vi "complexsignalpropogation.vi"() -> ()   [LabVIEW 2009]
uses:
  <vilib>/imath/engines/lvmath2/RunTimeEngine/ErrorHandling/NIMS_Finalize Error.vi
  <vilib>/imath/engines/lvmath2/RunTimeEngine/Parser/MC_Version.vi
  <vilib>/imath/engines/lvmath2/RunTimeEngine/Managers/WorkSpace/UID Generator.vi
  <vilib>/imath/engines/lvmath2/RunTimeEngine/NodeEndStatement/NIMS_NodeEndStatement_Output.vi
  <instcachedir>/0/NIMS_NodeEndStatement_Output_53EC0D466D134D7ABD903AC30B43404B.lvgen/NIMS_NodeEndStatement_Output_53EC0D466D134D7ABD903AC30B43404B_001.vi
  <vilib>/imath/engines/lvmath2/RunTimeEngine/NodeEndStatement/MC_NodeEndStatement_Dispose.vi
  <vilib>/imath/engines/lvmath/Functions/Error Handling/MergeErrorsWrapper.vi
  <vilib>/imathl/engines/lvmath/Functions/Error Handling/Create Error.vi
  <vilib>/imath/engines/lvmath2/RunTimeEngine/RunTimeType/NIMS_RunTimeType_Get Case Value.vi
  <vilib>/imath/engines/lvmath2/RunTimeEngine/Managers/SymbolTable/Read Variable.vi
  <vilib>/imath/engines/lvmath2/RunTimeEngine/CommandStatement/NIMS_CommandStatement_MaskErr.vi
  <vilib>/imath/engines/lvmath2/RunTimeEngine/Managers/SymbolTable/Write Variable.vi
  <vilib>/imath/engines/lvmath2/RunTimeEngine/ArithmeticOperatorToken/NIMS_NS_ArithmeticOperator_cctranspose.vi
  <vilib>/imath/engines/lvmath2/RunTimeEngine/RunTimeSymbolToken/NIMS_RunTimeSymbolToken_ReadVariable.vi
  <vilib>/imath/engines/lvmath2/RunTimeEngine/RangeToken/NIMS_NS_Range - 2 inputs.vi
  <vilib>/imath/engines/lvmath2/RunTimeEngine/RunTimeSymbolToken/NIMS_RunTimeSymbolToken_ResolveSymbol.vi
  <instcachedir>/0/NIMS_RunTimeSymbolToken_ResolveSymbol_94D143D0F28444E2BA7BB87D83E1A664.lvgen/NIMS_RunTimeSymbolToken_ResolveSymbol_94D143D0F28444E2BA7BB87D83E1A664_000.vi
  <vilib>/imath/engines/lvmath2/RunTimeEngine/ArithmeticOperatorToken/NIMS_NS_ArithmeticOperator_rightdivmx.vi
  <vilib>/imath/engines/lvmath2/RunTimeEngine/ArithmeticOperatorToken/NIMS_NS_ArithmeticOperator_multmx.vi
  <vilib>/imath/engines/lvmath2/RunTimeEngine/RangeToken/NIMS_NS_Range - 3 inputs.vi
  <vilib>/imath/engines/lvmath2/RunTimeEngine/ArithmeticOperatorToken/NIMS_NS_ArithmeticOperator_minus.vi
  <instcachedir>/0/NIMS_RunTimeSymbolToken_ResolveSymbol_94D143D0F28444E2BA7BB87D83E1A664.lvgen/NIMS_RunTimeSymbolToken_ResolveSymbol_94D143D0F28444E2BA7BB87D83E1A664_001.vi
  <vilib>/imath/engines/lvmath2/RunTimeEngine/NonStaticBuiltInFunctions/Manual/NIMS_NS_clear.vi
  <vilib>/imath/engines/lvmath2/RunTimeEngine/NonStaticBuiltInFunctions/NIMS_NS_cos.vi
  <vilib>/imath/engines/lvmath2/RunTimeEngine/NonStaticBuiltInFunctions/NIMS_NS_sin.vi
  <vilib>/imath/engines/lvmath2/RunTimeEngine/RunTimeType/NIMS_RunTimeType_From StrictType (excl LVString).vi
  <vilib>/imath/engines/lvmath2/RunTimeEngine/RunTimeType/NIMS_RunTimeType_To Numeric.vi
  <instcachedir>/0/NIMS_RunTimeType_To Numeric_461D4BB0B5AC4C7A80E516929E1870C9.lvgen/NIMS_RunTimeType_To Numeric_461D4BB0B5AC4C7A80E516929E1870C9_000.vi
  <vilib>/imath/engines/lvmath/Plug In/_Char/RunTimeType/NIMS_CH_RunTimeType_To Character 2D.vi
  <vilib>/imath/engines/lvmath/Plug In/_PlotObject/RunTimeType/NIMS_PO_RunTimeType_To Plot object 2D.vi
  <vilib>/imath/engines/lvmath2/RunTimeSupport/NIMS_Clear Errors.vi
  <vilib>/imath/engines/lvmath2/RunTimeEngine/ReplaceToken/NIMS_NS_Replace - M(M)=M.vi
  <vilib>/imath/engines/lvmath2/RunTimeEngine/LoopVariableIndexToken/NIMS_NS_LoopVariableIndexToken_Index.vi
  <vilib>/imath/engines/lvmath2/RunTimeEngine/CommandStatement/MC_CommandStatement_break.vi
  <vilib>/imath/engines/lvmath2/RunTimeEngine/NodeEndStatement/NIMS_NodeEndStatement_Get Vector.vi
  <instcachedir>/0/NIMS_NodeEndStatement_Get Vector_708AE642CFEE4B9892E482CBBBA3A4D6.lvgen/NIMS_NodeEndStatement_Get Vector_708AE642CFEE4B9892E482CBBBA3A4D6_001.vi
  <vilib>/imath/engines/lvmath/Plug In/_Char/NIMS_CH_Character 1D to U8 1D.vi
  <instcachedir>/0/NIMS_NodeEndStatement_Get Vector_708AE642CFEE4B9892E482CBBBA3A4D6.lvgen/NIMS_NodeEndStatement_Get Vector_708AE642CFEE4B9892E482CBBBA3A4D6_002.vi
  <vilib>/imath/engines/lvmath/Functions/Error Handling/error.ctl
  <vilib>/Platform/NI_3dgraph.lvlib
  <vilib>/imath/engines/lvmath2/RunTimeEngine/Managers/SymbolTable/NIMS_WorkSpace.lvlib
panel:
  in  "Spiral of cos(wt) + jsin(wt)":refnum<k7>(container)
  out "Real and Imag x":cluster{dbl[], dbl[]}[](graph)
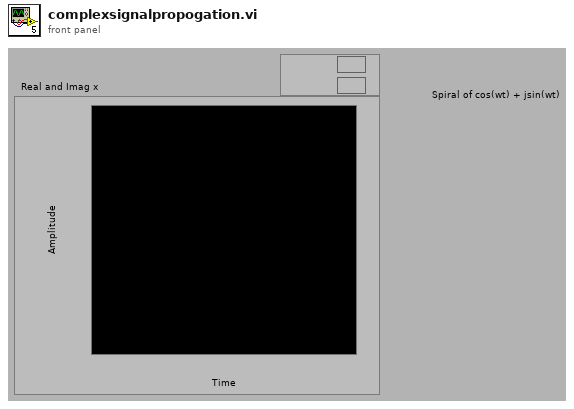
[diagram p1: front panel]
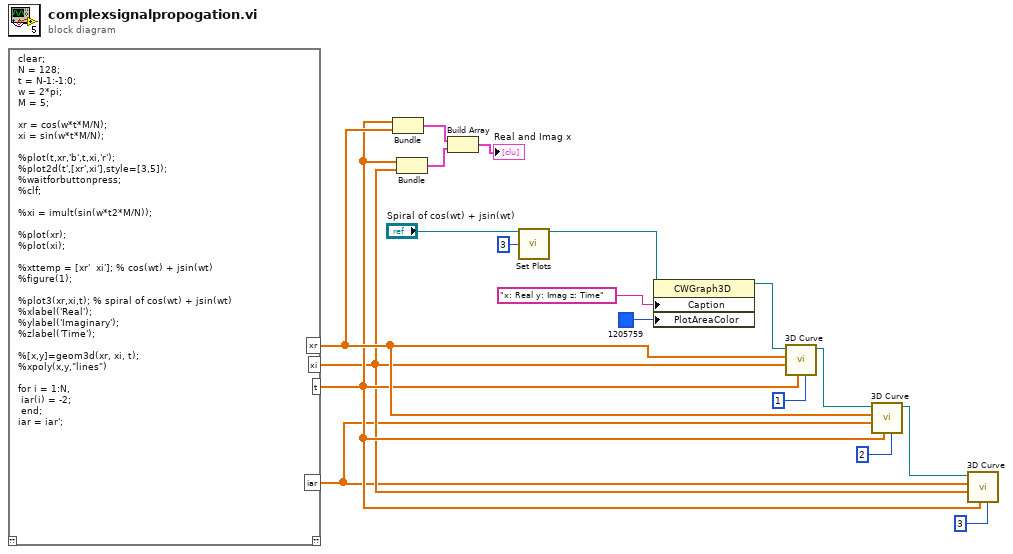
[diagram p0: block diagram]
diagram:
  n1 = mathscript code="clear;\nN = 128;\nt = N-1:-1:0;\nw = 2*pi;\nM = 5;\n\nxr = cos(w*t*M/N);\nxi = sin(w*t*M/N);\n\n%plot(t,xr,'b',t,xi,'r');\n%plot2d(t',[xr',xi'],style=[3,5]);\n%waitforbuttonpress;\n%clf;\n\n%xi = imult(sin(w*t2*M/N));\n\n%plot(xr);\n%plot(xi);\n\n%xttemp = [xr'  xi']; % cos(wt) + jsin(wt)\n%figure(1);\n\n%plot3(xr,xi,t); % spiral of cos(wt) + jsin(wt)\n%xlabel('Real');\n%ylabel('Imaginary');\n%zlabel('Time');\n\n%[x,y]=geom3d(xr, xi, t);\n%xpoly(x,y,\"lines\")\n\nfor i = 1:N,\n iar(i) = -2;\n end;\niar = iar';"() -> ("xr"=w15:dbl[], "xi"=w2:dbl[], "t"=w14:dbl[], "iar"=w1:dbl[])  [unwired: 1 in, 1 out]
  n2 = Bundle(w14, w15) -> (w18:cluster{dbl[], dbl[]})  [unwired: 1 in]
  n3 = Bundle(w14, w2) -> (w17:cluster{dbl[], dbl[]})  [unwired: 1 in]
  n4 = Build Array(w18, w17) -> (→"Real and Imag x":cluster{dbl[], dbl[]}[])
  n5 = call <vilib>:"Set Plots.vi"("3D graph"="Spiral of cos(wt) + jsin(wt)", "# of plots(1)"=3) -> ("3D graph out"=w9:refnum<k7>)  [unwired: 12 in, 1 out]
  n6 = property class="CWGraph3D"(reference=w9, "Caption"="x: Real y: Imag z: Time", "PlotAreaColor"=u32 1205759) -> (reference out=w8:refnum<k7>)  [unwired: 1 in, 1 out]
  n7 = call <vilib>:"3D Curve.vi"("plot number (1)"=1, "z vector"=w14, "y vector"=w2, "x vector"=w15, "3D graph"=w8) -> ("3D graph out"=w7:refnum<k7>)  [unwired: 5 in, 1 out]
  n8 = call <vilib>:"3D Curve.vi"("plot number (1)"=2, "z vector"=w14, "y vector"=w1, "x vector"=w15, "3D graph"=w7) -> ("3D graph out"=w6:refnum<k7>)  [unwired: 5 in, 1 out]
  n9 = call <vilib>:"3D Curve.vi"("plot number (1)"=3, "z vector"=w14, "y vector"=w2, "x vector"=w1, "3D graph"=w6) -> ()  [unwired: 5 in, 2 out]
